vi "Array 3.vi"() -> ()   [LabVIEW 2011]
panel:
  out "Array":dbl[](array[numeric])
  in  "Numeric 4":dbl
  in  "Numeric 2":dbl
  in  "Numeric 3":dbl
  in  "Numeric":dbl
  out "final output":dbl[](array[numeric])
  out "deleted portion":dbl[](array[numeric])
  in  "index":dbl
  in  "length":dbl
  in  "input array":dbl[](array[numeric])
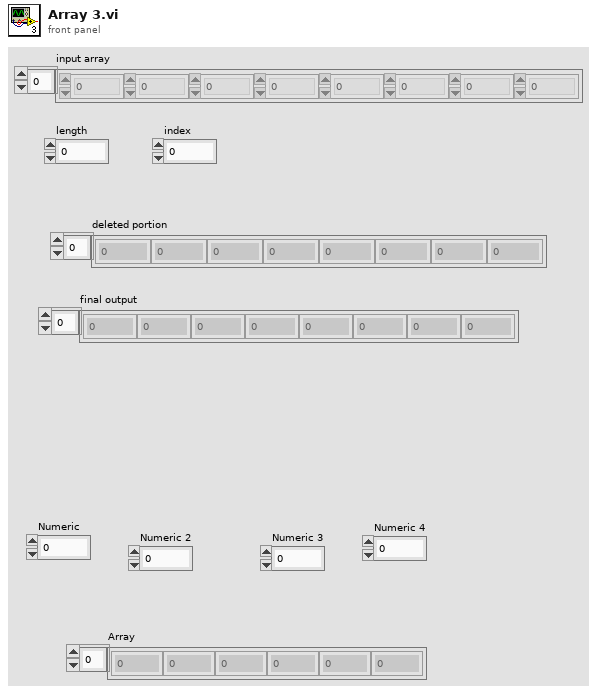
[diagram p1: front panel]
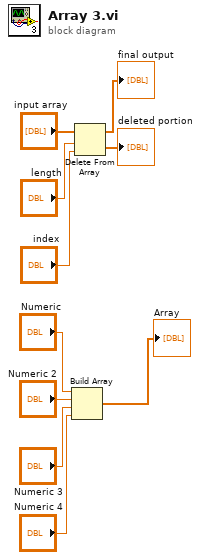
[diagram p0: block diagram]
diagram:
  n1 = Build Array("Numeric", "Numeric 2", "Numeric 3", "Numeric 4") -> (→"Array":dbl[])
  n2 = Delete From Array(array="input array", length="length", index="index") -> (deleted portion=→"deleted portion":dbl[], array with subset deleted=→"final output":dbl[])
